vi "Substitute Assembly Versions.vi"(8 "error in":errorcluster, 11 "config file path":path) -> (0 "error out":errorcluster)   [LabVIEW 2020, in "Template Tool.lvlib"]
uses:
  Template Tool.lvlib
  <vilib>/Utility/config.llb/Read Key (String).vi
  <vilib>/Utility/config.llb/NI_LVConfig.lvlib
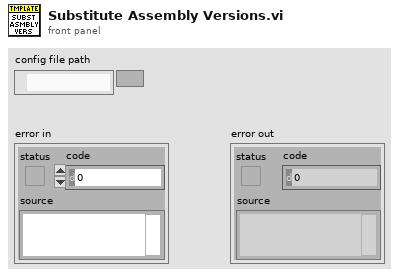
[diagram p1: front panel]
types:
  T1 = typedef "NI_LVConfig.lvlib/Config Data RefNum.ctl" = refnum<k1>
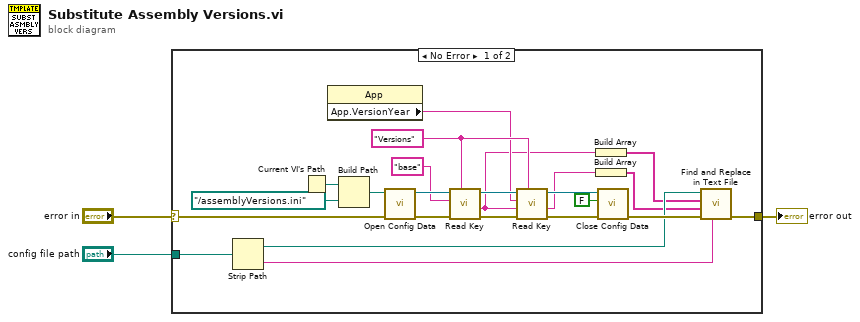
[diagram p0: block diagram]
diagram:
  n1 = case shown="No Error" "error in" {
    selector: "error in" -> [w19 w27]
    tunnel: [w10 w27] -> w3
    tunnel: "config file path" -> [w12 _]
    frame No Error {
      w16 = "Versions" ("section")
      n2 = Strip Path(path=w12) -> (stripped path=w8:path, name=w9:string)
      n3 = Current VI's Path() -> (path=w22:path)
      n4 = property class="App"() -> ("App.VersionYear"=w15:string)  [unwired: 2 in, 2 out]
      n5 = Build Path(base path=w22, name or relative path=path "../assemblyVersions.ini" ("configuration file path")) -> (appended path=w20:path)
      n6 = call <vilib>:"Open Config Data.vi"("error in (no error)"=w19, "configuration file path"=w20) -> ("error out"=w25:errorcluster, "refnum"=w24:T1)  [unwired: 7 in, 1 out]
      n7 = call-poly <vilib>:"Read Key.vi"("section"=w16, "error in (no error)"=w25, "key"="base", "refnum"=w24) -> ("error out"=w18:errorcluster, "value"=w7:string, "refnum out"=w17:T1)  [unwired: 4 in, 1 out]
      n8 = call-poly <vilib>:"Read Key.vi"("section"=w16, "error in (no error)"=w18, "default value"=w7, "key"=w15, "refnum"=w17) -> ("error out"=w14:errorcluster, "value"=w6:string, "refnum out"=w13:T1)  [unwired: 3 in, 1 out]
      n9 = Build Array(w7) -> (w5:string[])
      n10 = Build Array(w6) -> (w4:string[])
      n11 = call <vilib>:"Close Config Data.vi"("error in (no error)"=w14, "write file if changed (T)"=FALSE, "refnum"=w13) -> ("error out"=w11:errorcluster)  [unwired: 7 in, 1 out]
      n12 = call "Find and Replace in Text File.vi"("file name"=w9, "error in"=w11, "replace array"=w4, "find array"=w5, "folder path"=w8) -> ("error out"=w10:errorcluster)  [unwired: 5 in, 1 out]
    }
    frame Error {
    }
  }
  "error out" <- w3
